vi "USRP Google Maps Example.vi"() -> ()   [LabVIEW 2012]
uses:
  <vilib>/wsapi/NI_WebServices.lvlib
panel:
  out "Google URL (not escaped)":string
  out "Has GPS Disciplined Clock?":bool
  in  "GPS Fix Timeout":dbl=180.0
  in  "device names":refnum<k15>="192.168.10.2"
  in  "active antenna":string="RX1"
  out "coerced gain":dbl=10.0 format="%#_6f"
  out "coerced carrier frequency":dbl=315000000.0 format="%#_6p"
  out "coerced IQ rate":dbl=1000000.0 format="%#_6p"
  in  "gain":dbl=10.0 format="%#_6f"
  in  "carrier frequency":dbl=315000000.0 format="%#_6p"
  in  "IQ rate":dbl=1000000.0 format="%#_6p"
  out "GPS Time":timestamp=timestamp(3448974302.011462 s since 1904-01-01)
  out "GPS Disciplined Clock:GPS Sentence GGA":string
  in  "Map Type":string(combo)="roadmap"
  in  "Zoom Level":u8=14 max=21 step=1
  out "GPSDC:GPS Sentence RMC":string="$GPRMC,162500.00,A,3024.4895,N,09743.5488,W,0.0,0.0,160413,,*2D\r"
  out "error out":errorcluster
  in  "Map Width":i32=499
  in  "Map Height":i32=287
  in  "stop":bool
  in  "WebBrowser":refnum<k7>(container)
  # "Map Settings"
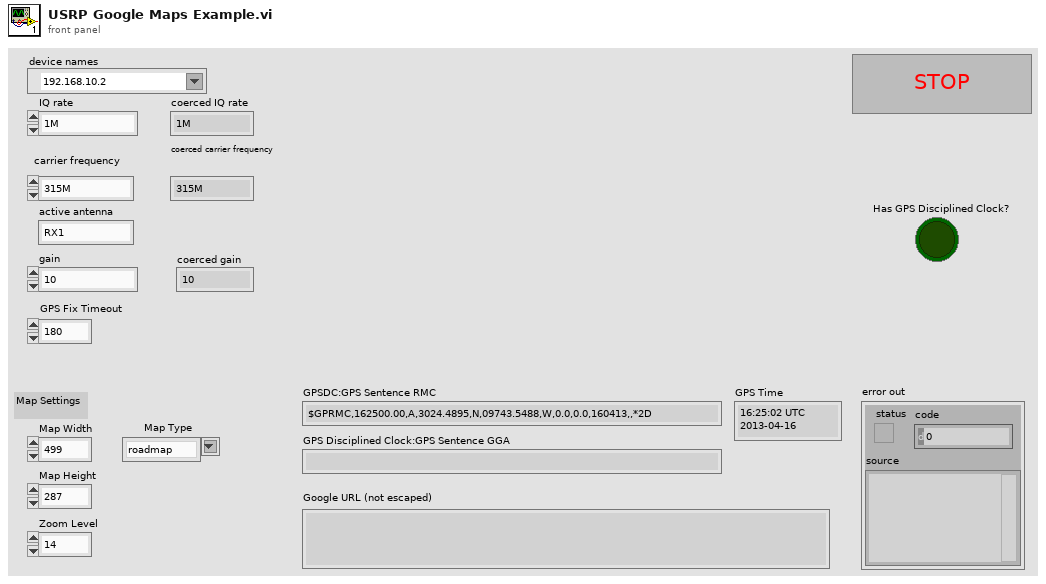
[diagram p1: front panel]
types:
  T1 = typedef "niUSRP Timestamp.ctl" = cluster{"whole seconds":u64, "fractional seconds":dbl}
  T2 = cluster{"Time Stamp":timestamp, "Latitude (ddmm.mmmm)":dbl, "Latitude North/South":string, "Longitude (dddmm.mmmm)":dbl, "Longitude East/West":string, "Magnetic Variation (degrees)":dbl, "Magnetic Variation East/West":string, "Speed over ground (knots)":dbl, "Course over ground (degrees)":dbl}
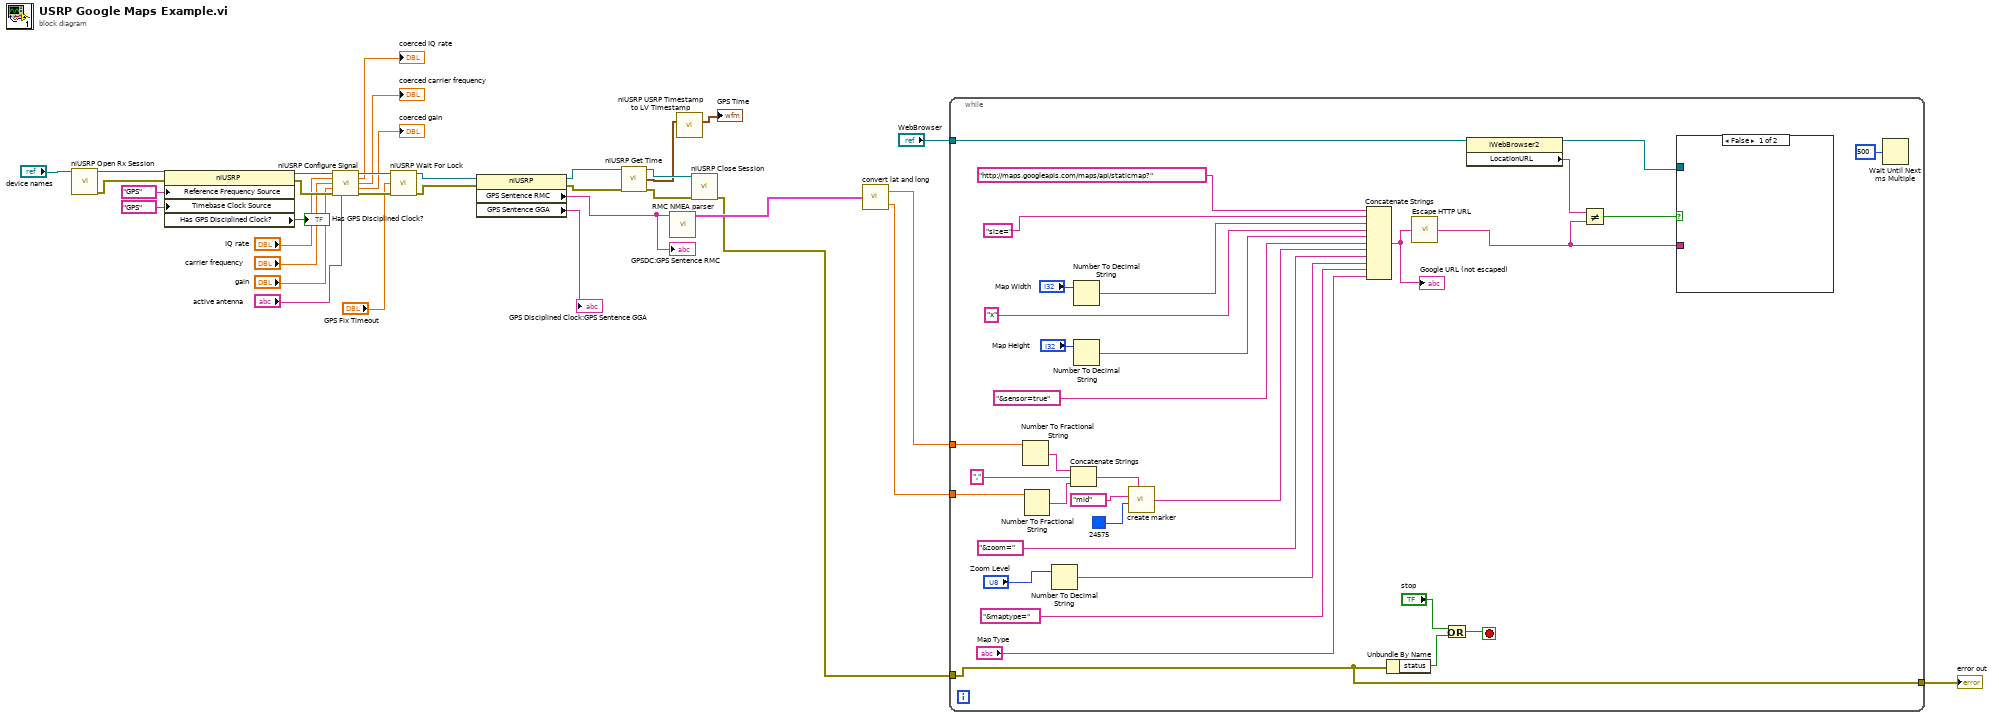
[diagram p0: block diagram]
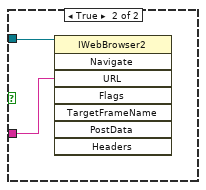
[diagram p2: hidden frame]
diagram:
  n1 = call <instrlib>:"niUSRP Open Rx Session.vi"("device names"="device names") -> ("session handle out"=w33:refnum<k15>, "error out"=w32:errorcluster)  [unwired: 13 in]
  n2 = property class="niUSRP"(reference=w33, error in=w32, "Reference Frequency Source"="GPS" ("Clocking and Synchronization:Reference Frequency Source"), "Timebase Clock Source"="GPS" ("Clocking and Synchronization:Timebase Clock Source")) -> (reference out=w29:refnum<k15>, error out=w28:errorcluster, "Has GPS Disciplined Clock?"=→"Has GPS Disciplined Clock?":bool)
  n3 = call <instrlib>:"niUSRP Configure Signal.vi"("session handle"=w29, "IQ rate"="IQ rate", "carrier frequency"="carrier frequency", "gain"="gain", "error in (no error)"=w28, "active antenna"="active antenna") -> ("session handle out"=w27:refnum<k15>, "coerced IQ rate"=→"coerced IQ rate":dbl, "coerced carrier frequency"=→"coerced carrier frequency":dbl, "coerced gain"=→"coerced gain":dbl, "error out"=w26:errorcluster)  [unwired: 5 in]
  n4 = call <instrlib>:"niUSRP Wait For Lock.vi"("session handle"=w27, "timeout"="GPS Fix Timeout", "error in (no error)"=w26) -> ("session handle out"=w24:refnum<k15>, "error out"=w23:errorcluster)  [unwired: 11 in]
  n5 = property class="niUSRP"(reference=w24, error in=w23) -> (reference out=w17:refnum<k15>, error out=w16:errorcluster, "GPS Sentence RMC"=w18:string, "GPS Sentence GGA"=→"GPS Disciplined Clock:GPS Sentence GGA":string)
  "GPSDC:GPS Sentence RMC" <- w18
  n6 = call <instrlib>:"niUSRP Get Time.vi"("session handle"=w17, "error in (no error)"=w16) -> ("session handle out"=w14:refnum<k15>, "USRP Timestamp"=w13:T1, "error out"=w15:errorcluster)  [unwired: 11 in]
  n7 = call "RMC NMEA parser.vi"("RMC String"=w18) -> ("GPS Data"=w22:T2)  [unwired: 9 in, 1 out]
  n8 = call <instrlib>:"niUSRP USRP Timestamp to LV Timestamp.vi"("USRP Timestamp"=w13) -> ("LV Timestamp"=→"GPS Time":timestamp)  [unwired: 13 in, 1 out]
  n9 = call <instrlib>:"niUSRP Close Session.vi"("session handle"=w14, "error in (no error)"=w15) -> ("error out"=w3:errorcluster)  [unwired: 13 in]
  n10 = call "convert lat and long.vi"("GPS Data"=w22) -> ("Latitude"=w21:dbl, "Longtitude"=w20:dbl)  [unwired: 4 in]
  n11 = while {
    tunnel: "WebBrowser" -> [w67]
    tunnel: w21 -> [w55]
    tunnel: w20 -> [w54]
    tunnel: w3 -> [w35]
    tunnel: [w35] -> w2
    stop <- w38 stop-if-true
    n12 = Number To Fractional String(number=w55) -> (F-format string=w53:string)  [unwired: 3 in]
    n13 = Number To Fractional String(number=w54) -> (F-format string=w51:string)  [unwired: 3 in]
    n14 = Number To Decimal String(number="Zoom Level") -> (decimal integer string=w43:string)  [unwired: 1 in]
    n15 = Concatenate Strings(w53, ",", w51) -> (w50:string)
    n16 = Number To Decimal String(number="Map Width") -> (decimal integer string=w60:string)  [unwired: 1 in]
    n17 = Number To Decimal String(number="Map Height") -> (decimal integer string=w58:string)  [unwired: 1 in]
    n18 = call "create marker.vi"("Location"=w50, "Color"=u32 24575, "Size"="mid") -> ("Marker String"=w49:string)  [unwired: 3 in]
    n19 = Concatenate Strings("http://maps.googleapis.com/maps/api/staticmap?", "size=", w60, "x", w58, "&sensor=true", w49, "&zoom=", w43, "&maptype=", "Map Type") -> (w47:string)
    "Google URL (not escaped)" <- w47
    n20 = Unbundle By Name(w35) -> ("status"=w37:bool)
    n21 = call <vilib>:"Escape HTTP URL.vi"("unescaped string in"=w47) -> ("escaped string out"=w40:string)
    n22 = Or(x="stop", y=w37) -> (x .or. y?=w38:bool)
    n23 = property class="IWebBrowser2"(reference=w67) -> (reference out=w64:refnum<k7>, "LocationURL"=w66:string)  [unwired: 1 in, 1 out]
    n24 = Not Equal?(x=w66, y=w40) -> (x != y?=w39:bool)
    n25 = case shown="False" w39 {
      tunnel: w40 -> [_ w69]
      tunnel: w64 -> [_ w68]
      frame False {
      }
      frame True {
        n26 = invoke class="IWebBrowser2" method="Navigate"(reference=w68, "URL"=w69) -> ()  [unwired: 6 in, 8 out]
      }
    }
    n27 = Wait Until Next ms Multiple(millisecond multiple=u32 500) -> ()  [unwired: 1 out]
  }
  "error out" <- w2
